vi "FurnaceControl_ME.vi"(0 "StoichTemp":dbl format="%#_13g", 1 "Stoich Array":dbl[](array[numeric])=[0.0], 2 "Target Temp":dbl, 3 "Furnace Setpoint":dbl format="%#_13g", 4 "Previous Setpoint":dbl format="%#_13g", 5 "User Setpoint":dbl format="%#_13g", 6 "Auto Change":string[][](array[string])=[["Timestamp", "Actual T", "Target T", "Delta T", "Previous Sp", "New Sp"]], 7 "Countdown":i32, 8 "User Change":string[][](array[string])=[["Timestamp", "Actual T", "Target T", "Previous Sp", "New Sp"]]) -> (10 "UserChanges":string[][](table), 12 "AutoChanges":string[][](table), 14 "Furnace Setpoint":dbl format="%#_13g", 15 "User Setpoint":dbl format="%#_13g", 16 "Stoich Array":dbl[](array[numeric]), 17 "countdown":i32, 18 "Limit Exceeded":bool)   [LabVIEW 2014]
uses:
  <vilib>/Analysis/baseanly.llb/Mean (DBL).vi
  <vilib>/Analysis/NI_AALBase.lvlib
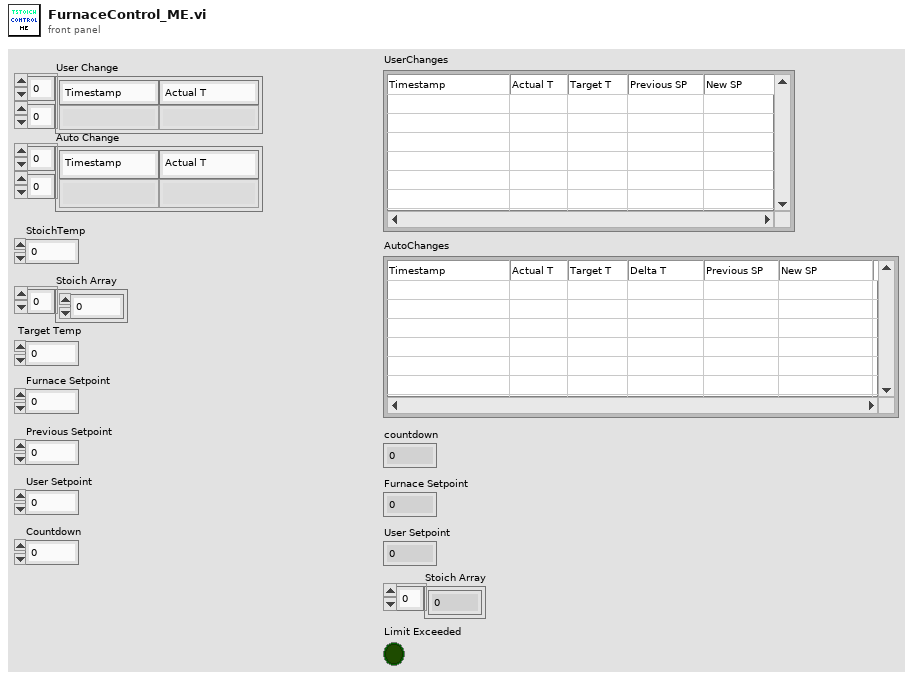
[diagram p1: front panel]
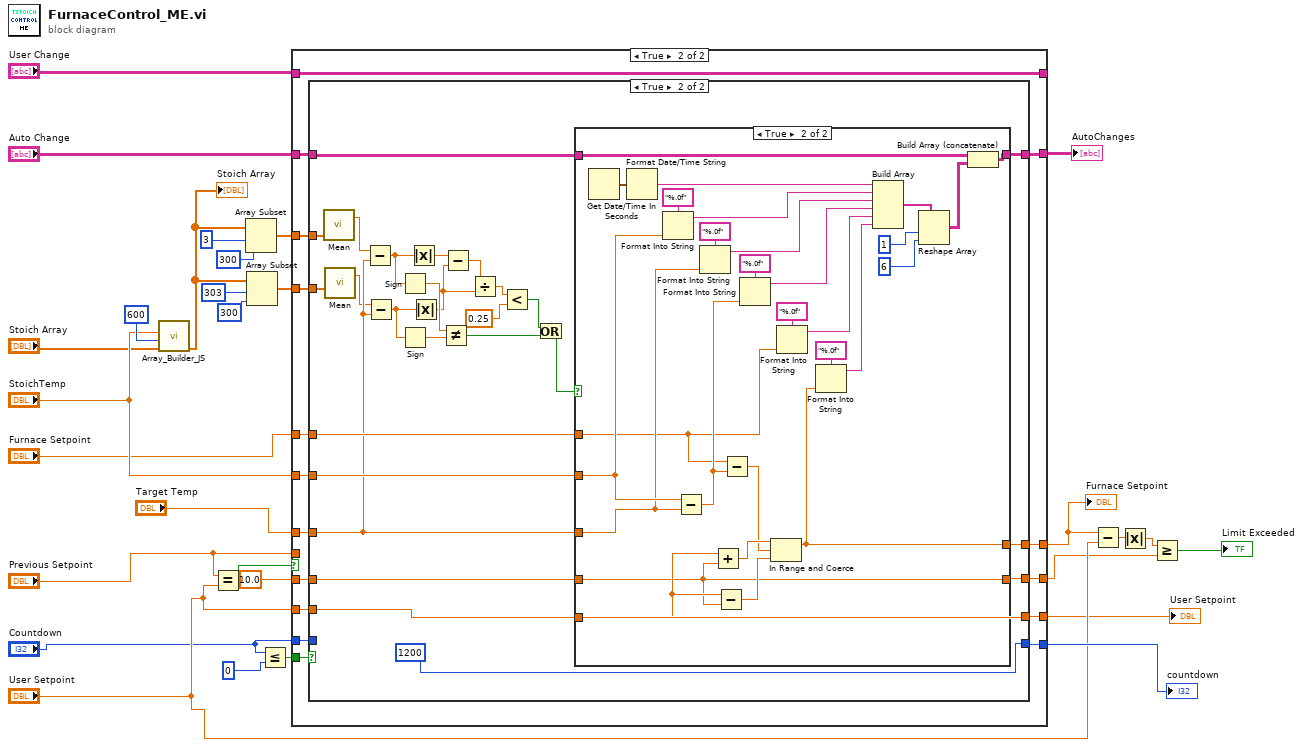
[diagram p0: block diagram]
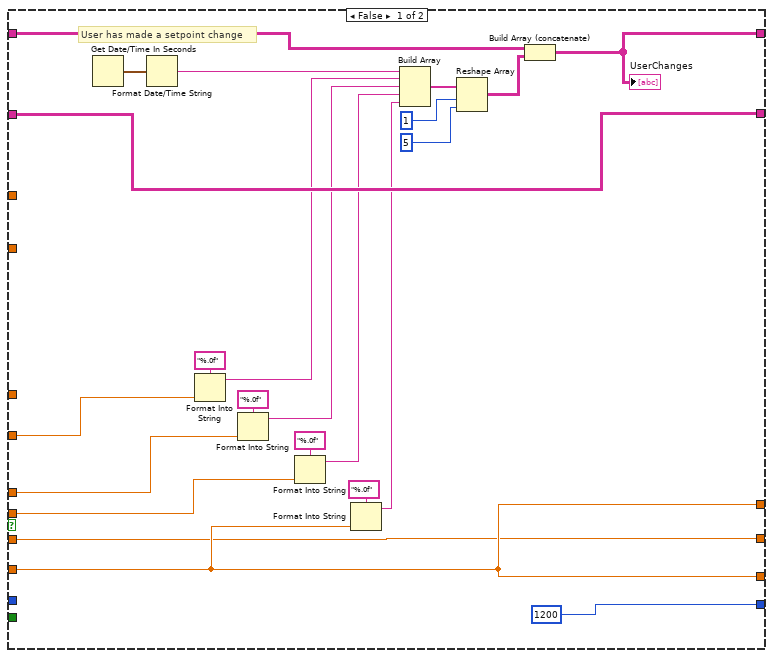
[diagram p2: hidden frame]
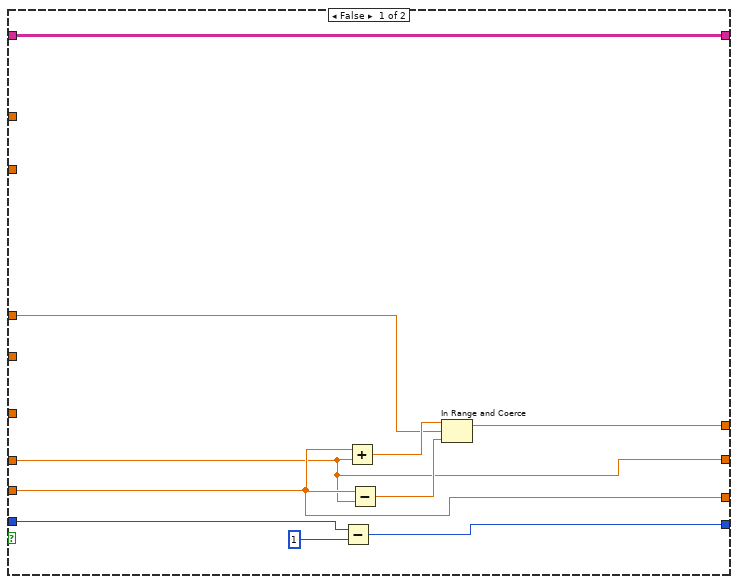
[diagram p3: hidden frame]
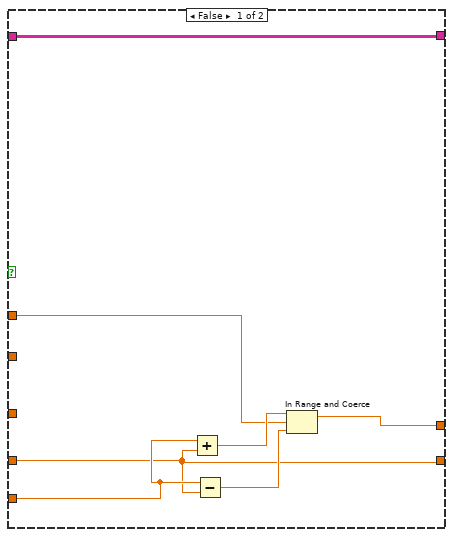
[diagram p4: hidden frame]
diagram:
  n1 = call "Array_Builder_JS.vi"("Array In"="Stoich Array", "Cycle Length"=600, "Input"="StoichTemp") -> ("Array Out Main"=w1:dbl[])  [unwired: 7 in, 1 out]
  "Stoich Array" <- w1
  n2 = Equal?(x="Previous Setpoint", y="User Setpoint") -> (x = y?=w25:bool)
  n3 = Array Subset(array=w1, index=3, length=300) -> (w17:dbl[])
  n4 = Array Subset(array=w1, index=303, length=300) -> (w18:dbl[])
  n5 = Less Or Equal?(x="Countdown", y=0) -> (x <= y?=w28:bool)
  n6 = case shown="True" w25 {
    tunnel: w28 -> [_ w68]
    tunnel: "Countdown" -> [_ w67]
    tunnel: [1200 ("Settling Time") w66] -> w24
    tunnel: "StoichTemp" -> [w44 w65]
    tunnel: "Target Temp" -> [w46 w64]
    tunnel: "User Setpoint" -> [w50 w63]
    tunnel: "Furnace Setpoint" -> [_ w62]
    tunnel: [w50 w61] -> w13
    tunnel: 10.0 -> [w30 w60]
    tunnel: [w50 w59] -> w6
    tunnel: "Previous Setpoint" -> [w47 _]
    tunnel: "User Change" -> [w32 w57]
    tunnel: "Auto Change" -> [w43 w58]
    tunnel: [w43 w56] -> w16
    tunnel: [w31 w57] -> _
    tunnel: w18 -> [_ w54]
    tunnel: w17 -> [_ w55]
    tunnel: [w30 w53] -> w10
    frame False {
      # "User has made a setpoint change"
      n7 = Get Date/Time In Seconds() -> (seconds since 1Jan1904=w52:timestamp)
      n8 = Format Date/Time String(seconds (now)=w52) -> (date/time string=w41:string)  [unwired: 2 in]
      n9 = Format Into String(format string="%.0f", w44) -> (resulting string=w40:string)  [unwired: 2 in, 1 out]
      n10 = Format Into String(format string="%.0f", w46) -> (resulting string=w39:string)  [unwired: 2 in, 1 out]
      n11 = Format Into String(format string="%.0f", w47) -> (resulting string=w38:string)  [unwired: 2 in, 1 out]
      n12 = Format Into String(format string="%.0f", w50) -> (resulting string=w37:string)  [unwired: 2 in, 1 out]
      n13 = Build Array(w41, w40, w39, w38, w37) -> (w36:string[])
      n14 = Reshape Array(w36, 1 ("Settling Time"), 5 ("Settling Time")) -> (w33:string[][])
      n15 = Build Array (concatenate)(w32, w33) -> (w31:string[][])
      "UserChanges" <- w31
    }
    frame True {
      n16 = case shown="True" w68 {
        tunnel: w67 -> [w77 _]
        tunnel: [w76 1200] -> w66
        tunnel: w65 -> [_ w100]
        tunnel: w64 -> [_ w97]
        tunnel: w63 -> [w71 w103]
        tunnel: w62 -> [w73 w99]
        tunnel: [w72 w98] -> w61
        tunnel: w60 -> [w69 w104]
        tunnel: [w71 w103] -> w59
        tunnel: w58 -> [w70 w101]
        tunnel: [w70 w102] -> w56
        tunnel: w55 -> [_ w96]
        tunnel: w54 -> [_ w94]
        tunnel: [w69 w79] -> w53
        frame False {
          n17 = Subtract(x=w77, y=1) -> (x-y=w76:i32)
          n18 = Add(x=w71, y=w69) -> (x+y=w75:dbl)
          n19 = Subtract(x=w71, y=w69) -> (x-y=w74:dbl)
          n20 = In Range and Coerce(upper limit=w75, x=w73, lower limit=w74) -> (coerced(x)=w72:dbl)  [unwired: 1 out]
        }
        frame True {
          n21 = call-poly <vilib>:"Mean.vi"("X"=w96) -> ("mean"=w95:dbl)  [unwired: 1 out]
          n22 = call-poly <vilib>:"Mean.vi"("X"=w94) -> ("mean"=w93:dbl)  [unwired: 1 out]
          n23 = Subtract(x=w95, y=w97) -> (x-y=w92:dbl)
          n24 = Subtract(x=w93, y=w97) -> (x-y=w91:dbl)
          n25 = Sign(1:w92) -> (0:w89:dbl)
          n26 = Sign(1:w91) -> (0:w90:dbl)
          n27 = Absolute Value(x=w92) -> (abs(x)=w85:dbl)
          n28 = Absolute Value(x=w91) -> (abs(x)=w83:dbl)
          n29 = Not Equal?(x=w89, y=w90) -> (x != y?=w88:bool)
          n30 = Subtract(x=w85, y=w83) -> (x-y=w84:dbl)
          n31 = Divide(x=w84, y=w83) -> (x/y=w82:dbl)
          n32 = Less?(x=w82, y=0.25) -> (x < y?=w81:bool)
          n33 = Or(x=w81, y=w88) -> (x .or. y?=w87:bool)
          n34 = case shown="True" w87 {
            tunnel: w104 -> [w105 w112]
            tunnel: w103 -> [w107 w114]
            tunnel: [w106 w136] -> w102
            tunnel: w101 -> [w106 w135]
            tunnel: w100 -> [_ w133]
            tunnel: w97 -> [_ w128]
            tunnel: w99 -> [w108 w113]
            tunnel: [w109 w127] -> w98
            tunnel: [w105 w112] -> w79
            frame False {
              n35 = Add(x=w107, y=w105) -> (x+y=w111:dbl)
              n36 = Subtract(x=w107, y=w105) -> (x-y=w110:dbl)
              n37 = In Range and Coerce(upper limit=w111, x=w108, lower limit=w110) -> (coerced(x)=w109:dbl)  [unwired: 1 out]
            }
            frame True {
              n38 = Get Date/Time In Seconds() -> (seconds since 1Jan1904=w134:timestamp)
              n39 = Format Date/Time String(seconds (now)=w134) -> (date/time string=w121:string)  [unwired: 2 in]
              n40 = Format Into String(format string="%.0f", w133) -> (resulting string=w120:string)  [unwired: 2 in, 1 out]
              n41 = Subtract(x=w133, y=w128) -> (x-y=w125:dbl)
              n42 = Format Into String(format string="%.0f", w128) -> (resulting string=w119:string)  [unwired: 2 in, 1 out]
              n43 = Add(x=w114, y=w112) -> (x+y=w139:dbl)
              n44 = Subtract(x=w114, y=w112) -> (x-y=w138:dbl)
              n45 = Subtract(x=w113, y=w125) -> (x-y=w137:dbl)
              n46 = Format Into String(format string="%.0f", w125) -> (resulting string=w118:string)  [unwired: 2 in, 1 out]
              n47 = In Range and Coerce(upper limit=w139, x=w137, lower limit=w138) -> (coerced(x)=w127:dbl)  [unwired: 1 out]
              n48 = Format Into String(format string="%.0f", w113) -> (resulting string=w117:string)  [unwired: 2 in, 1 out]
              n49 = Format Into String(format string="%.0f", w127) -> (resulting string=w116:string)  [unwired: 2 in, 1 out]
              n50 = Build Array(w121, w120, w119, w118, w117, w116) -> (w124:string[])
              n51 = Reshape Array(w124, 1 ("Settling Time"), 6 ("Settling Time")) -> (w115:string[][])
              n52 = Build Array (concatenate)(w135, w115) -> (w136:string[][])
            }
          }
        }
      }
    }
  }
  "Furnace Setpoint" <- w13
  "countdown" <- w24
  "AutoChanges" <- w16
  "User Setpoint" <- w6
  n53 = Subtract(x=w13, y="User Setpoint") -> (x-y=w14:dbl)
  n54 = Absolute Value(x=w14) -> (abs(x)=w11:dbl)
  n55 = Greater Or Equal?(x=w11, y=w10) -> (x >= y?=→"Limit Exceeded":bool)
